vi "Run Test (LibraryRefnum).vi"(4 "timeout (2000 ms)":i32=2000, 5 "Test Report":refnum<class "Test Report.lvclass">, 6 "Verbose":bool, 7 "Report Path":path, 8 "error in":errorcluster, 10 "Library Refnum":refnum<vi>, 11 "Interactive (T)":bool=TRUE) -> (0 "error out":errorcluster, 3 "Test Results":refnum<class "Test Result.lvclass">)   [LabVIEW 2020, in "Caraya.lvlib"]
doc: "\"Run Tests\" from a preject reference:\n- Dynamically discovers Caraya unit tests and runs them\n- Outputs results in a UI ans/or Test Report (J-Unit or text)\n\n(Not compatible with RT targets or RunTime Engine)"
uses:
  Caraya.lvlib
  classes/Test Report/Test Report.lvclass
  classes/Test Result/Test Result.lvclass
  classes/Test Runner.Library/Test Runner.Library.lvclass
  C:/projects/caraya/src/classes/Test Runner/Test Runner.lvclass
  classes/Test Runner/Test Runner.lvclass
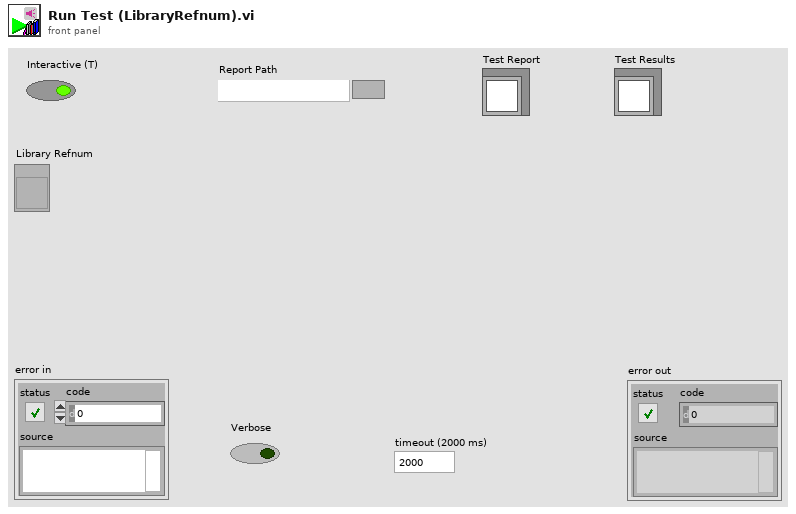
[diagram p1: front panel]
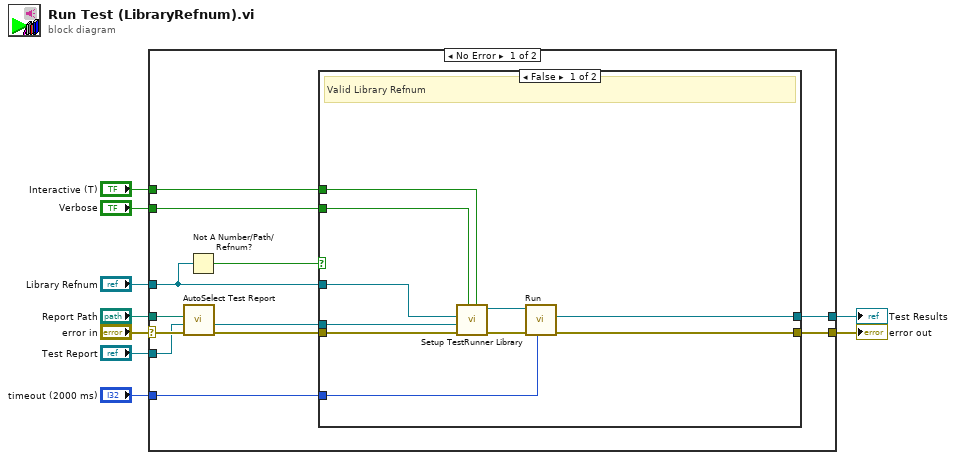
[diagram p0: block diagram]
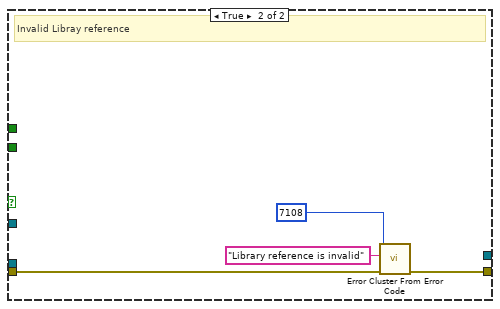
[diagram p2: hidden frame]
diagram:
  n1 = case shown="No Error" "error in" {
    selector: "error in" -> [w18 w36]
    tunnel: [w21 w36] -> w9
    tunnel: "Verbose" -> [w20 _]
    tunnel: "Interactive (T)" -> [w19 _]
    tunnel: "Test Report" -> [w15 _]
    tunnel: "Library Refnum" -> [w13 _]
    tunnel: "Report Path" -> [w17 _]
    tunnel: "timeout (2000 ms)" -> [w11 _]
    tunnel: [w10 _] -> w1
    frame No Error {
      n2 = call "AutoSelect Test Report.vi"("error in (no error)"=w18, "Test Report in"=w15, "Report Path"=w17) -> ("error out"=w16:errorcluster, "Test Report out"=w14:refnum<class "Test Report.lvclass">)  [unwired: 7 in]
      n3 = Not A Number/Path/Refnum?(number/path/refnum=w13) -> (NaN/Path/Refnum?=w12:bool)
      n4 = case shown="False" w12 {
        tunnel: [w31 w34] -> w21
        tunnel: w20 -> [w30 _]
        tunnel: w19 -> [w29 _]
        tunnel: w16 -> [w26 w35]
        tunnel: w14 -> [w25 _]
        tunnel: w13 -> [w24 _]
        tunnel: w11 -> [w23 _]
        tunnel: [w22 _] -> w10
        frame False {
          # "Valid Library Refnum"
          n5 = call "Setup TestRunner Library.vi"("Interactive (T)"=w29, "Verbose (F)"=w30, "error in (no error)"=w26, "Test Report"=w25, "Library Refnum"=w24) -> ("error out"=w27:errorcluster, "Test Runner.Library out"=w28:refnum<class "Test Runner.Library.lvclass">)  [unwired: 5 in]
          n6 = call "Run.vi"("timeout"=w23, "error in (no error)"=w27, "Test Runner in"=w28) -> ("error out"=w31:errorcluster, "Test Suite Results"=w22:refnum<class "Test Result.lvclass">)  [unwired: 6 in, 1 out]
        }
        frame True {
          # "Invalid Libray reference"
          n7 = call <vilib>:"Error Cluster From Error Code.vi"("error in (no error)"=w35, "error message (\"\")"="Library reference is invalid" ("error message (\"\")"), "error code (0)"=7108 ("code")) -> ("error out"=w34:errorcluster)  [unwired: 6 in]
        }
      }
    }
    frame Error {
    }
  }
  "error out" <- w9
  "Test Results" <- w1
